vi "Validate Error_Log_Folder.vi"(8 "Error In":errorcluster, 11 "Error_Log_Folder (string)":string) -> (0 "Error Out":errorcluster, 3 "Error_Log_Folder (path)":path)   [LabVIEW 2016, in "Error Manager.lvlib" / "Settings.lvclass"]
doc: "This VI performs one or more validation checks on the <B>Error_Log_Folder</B> setting value read from file.\n\nError Behaviour\n1. The VI skips execution if \"Error In\" contains an error. The input error is passed-through unaltered.\n2. If all validation checks passed the VI outputs \"No Error\".\n3. If a validation check failed the VI outputs an error with an informative error message."
uses:
  Settings.lvclass
  Error Manager.lvlib
  <vilib>/Utility/error.llb/whitespace.ctl
panel:
  # "Development\nControls or indicators that are useful for development or testing, but which are not outputs of the VI."
  # "Input\nInputs to the VI"
  # "Output\nOutputs of the VI"
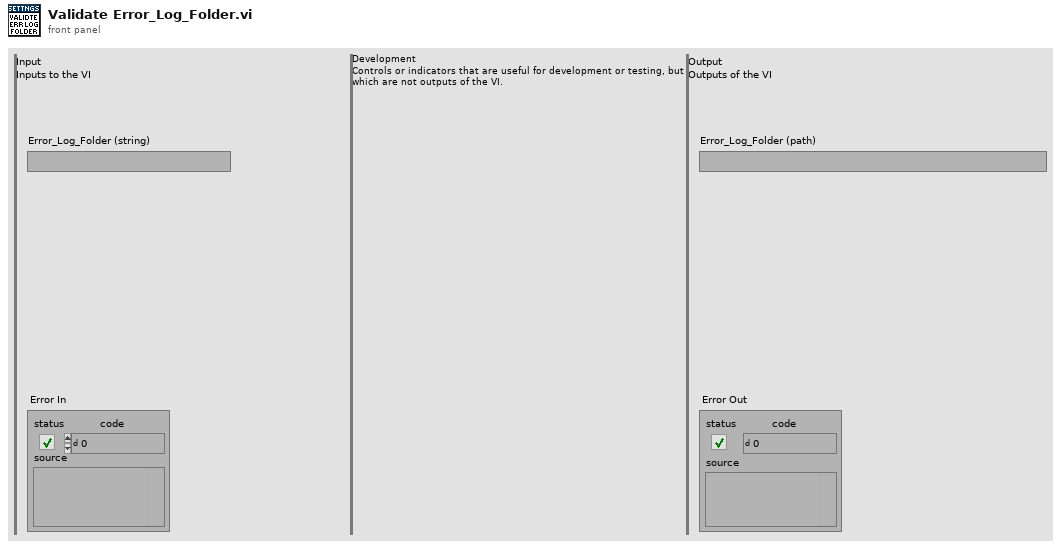
[diagram p1: front panel]
types:
  T1 = typedef "whitespace.ctl" = u16
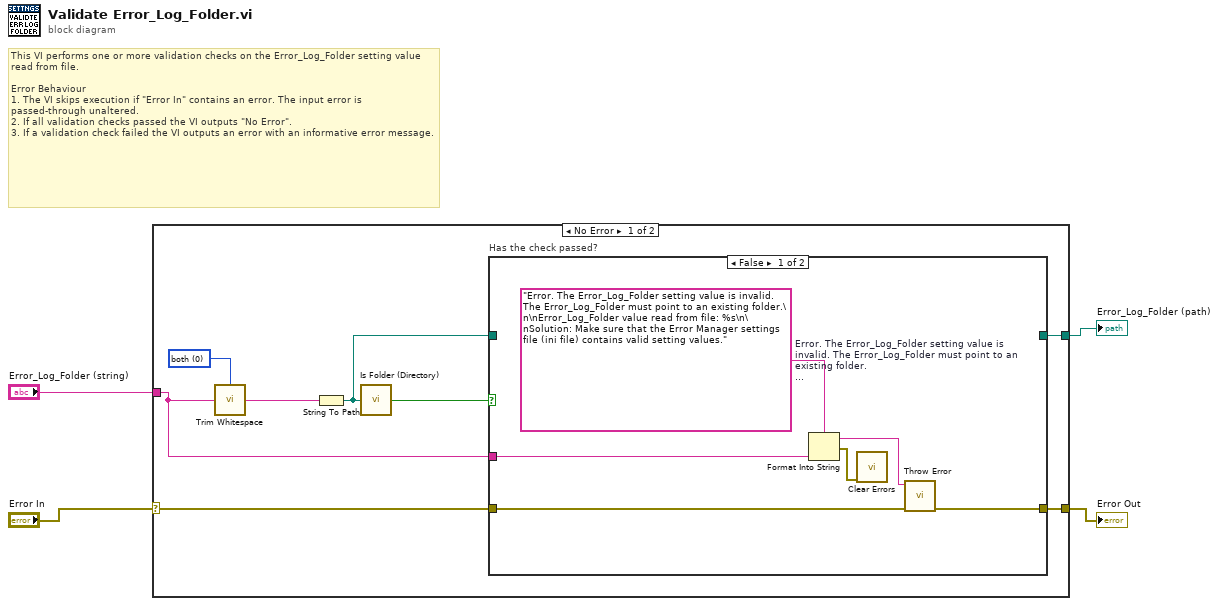
[diagram p0: block diagram]
diagram:
  # "This VI performs one or more validation checks on the Error_Log_Folder setting value read from file.\n\nError Behaviour\n1. The VI skips execution if \"Error In\" contains an error. The input error is passed-through unaltered.\n2. If all validation checks passed the VI outputs \"No Error\".\n3. If a validation check failed the VI outputs an error with an informative error message."
  n1 = case shown="No Error" "Error In" {
    selector: "Error In" -> [w12 w21]
    tunnel: [w11 w21] -> w3
    tunnel: "Error_Log_Folder (string)" -> [w7 _]
    tunnel: [w9 _] -> w1
    frame No Error {
      w5 = T1 0 items=["both", "start of string", "end of string"] ("location (both)")
      n2 = call <vilib>:"Trim Whitespace.vi"("string"=w7, "location (both)"=w5) -> ("trimmed string"=w6:string)
      n3 = String To Path(string=w6) -> (path=w8:path)
      n4 = call "Is Folder (Directory).vi"("Input Path"=w8) -> ("Is Folder?"=w10:bool)
      n5 = case "Has the check passed?" shown="False" w10 {
        tunnel: w12 -> [w18 w20]
        tunnel: [w17 w20] -> w11
        tunnel: [_ w19] -> w9
        tunnel: w8 -> [_ w19]
        tunnel: w7 -> [w13 _]
        frame False {
          w14 = "Error. The Error_Log_Folder setting value is invalid. The Error_Log_Folder must point to an existing folder.\n\nError_Log_Folder value read from file: %s\n\nSolution: Make sure that the Error Manager settings file (ini file) contains valid setting values."  # Error. The Error_Log_Folder setting value is invalid. The Error_Log_Folder must point to an existing folder.  Error_Log_Folder value read from file: %s  Solution: Make sure that the Error Manager settings file (ini file) contains valid setting values.
          n6 = Format Into String(format string=w14, w13) -> (resulting string=w15:string, error out=w16:errorcluster)  [unwired: 2 in]
          n7 = call <vilib>:"Clear Errors.vi"("error in (no error)"=w16) -> ()  [unwired: 5 in, 2 out]
          n8 = call "Throw Error.vi"("error in"=w18, "Error Message"=w15) -> ("error out"=w17:errorcluster)  [unwired: 9 in]
        }
        frame True {
        }
      }
    }
    frame Error {
    }
  }
  "Error Out" <- w3
  "Error_Log_Folder (path)" <- w1
